vi "Watlow Modbus.vi"(6 "Watlow Present?":bool, 7 "Modbus Mode":T2, 8 "Error IN":errorcluster, 10 "Data Write":sgl format="%#_13g", 11 "Variable":T1) -> (0 "Error OUT":errorcluster, 3 "Data Read":sgl)   [LabVIEW 2019]
uses:
  Modbus Mode.ctl
  Modbus Variable.ctl
  NI Modbus.llb/MB Modbus Command.ctl
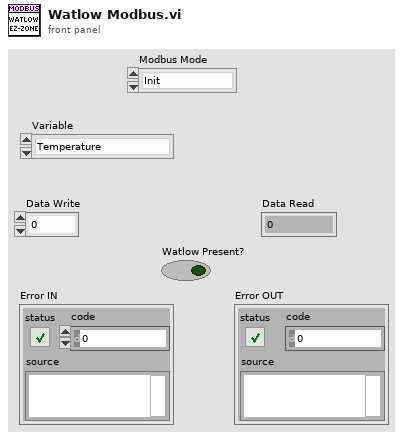
[diagram p1: front panel]
types:
  T1 = typedef "Modbus Variable.ctl" = enum16{"Temperature", "Setpoint"}
  T2 = typedef "Modbus Mode.ctl" = enum16{"Init", "Tank 1 Write", "Tank 2 Write", "Tank 1 Read", "Tank 2 Read", "F4T Write", "F4T Read"}
  T3 = cluster{"Mode":enum16{"RTU", "ASCII"}, "Slave Address":u8}
  T4 = typedef "MB Modbus Command.ctl" = cluster{"Function Code":u8, "Starting Address":u16, "Quantity":u16, "Data":u16[], "Discrete":bool[]}
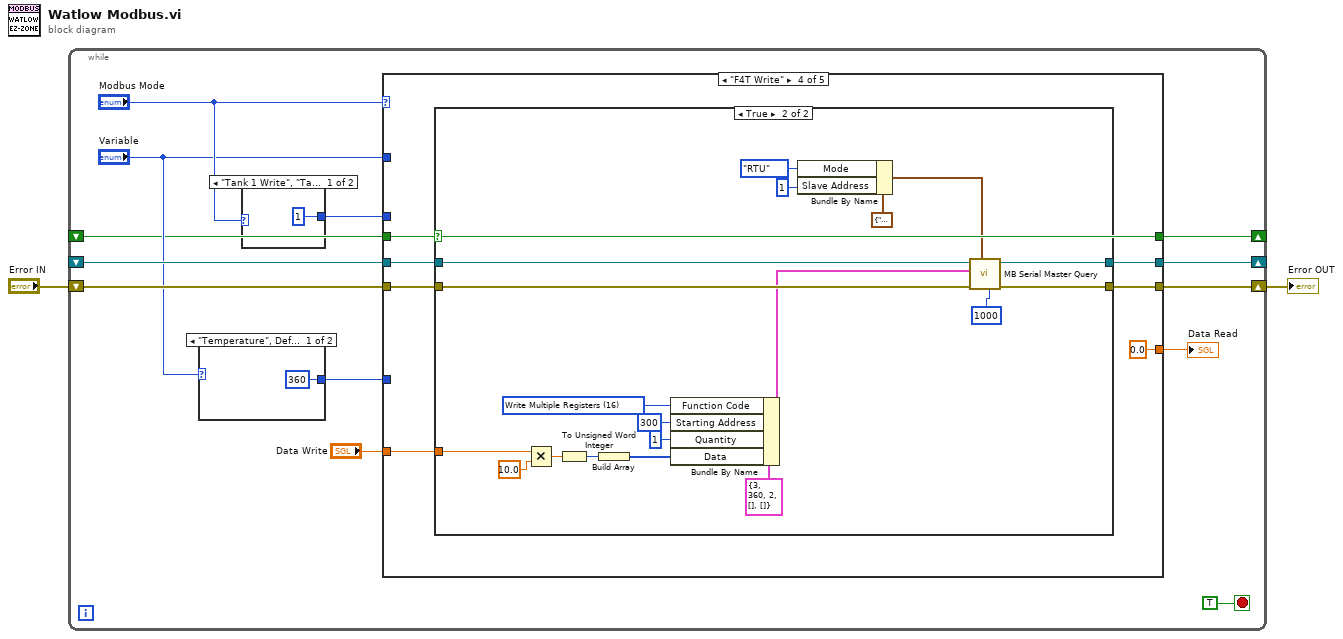
[diagram p0: block diagram]
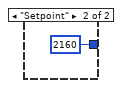
[diagram p2: hidden frame]
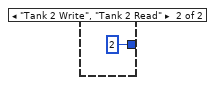
[diagram p3: hidden frame]
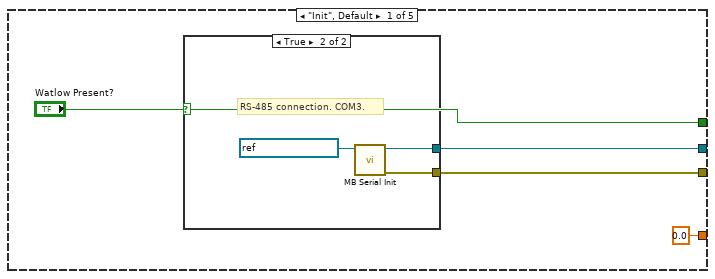
[diagram p4: hidden frame]
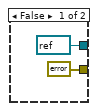
[diagram p5: hidden frame]
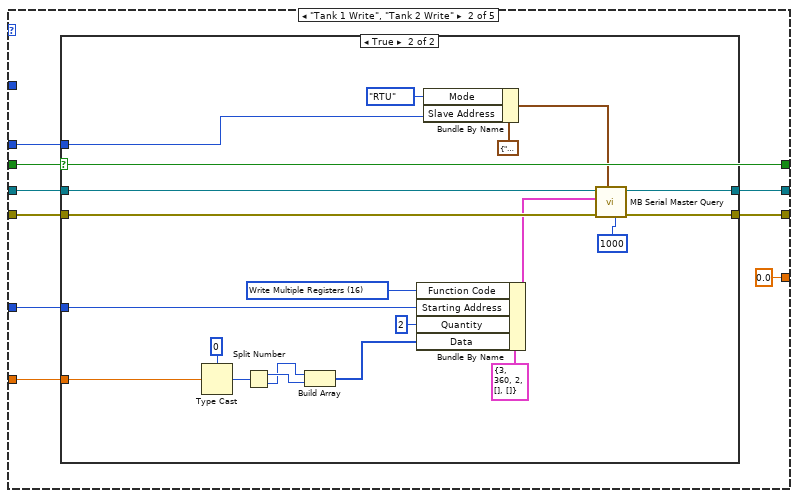
[diagram p6: hidden frame]
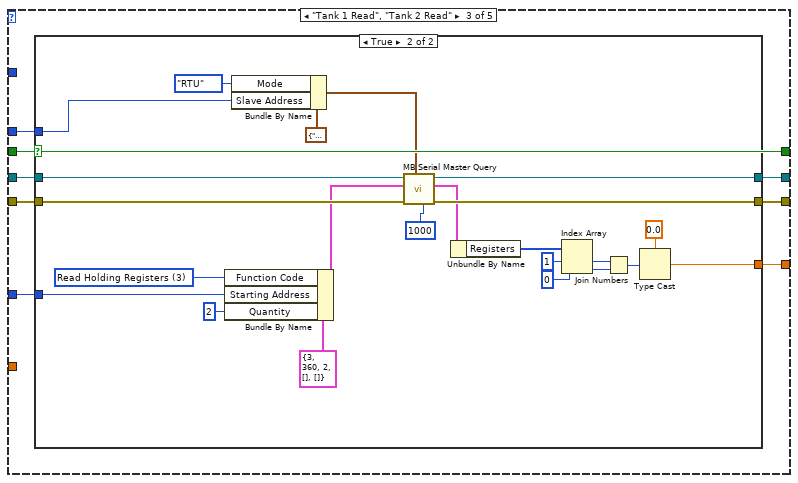
[diagram p8: hidden frame]
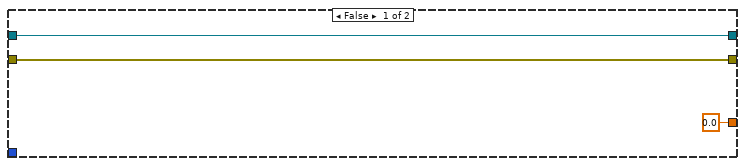
[diagram p9: hidden frame]
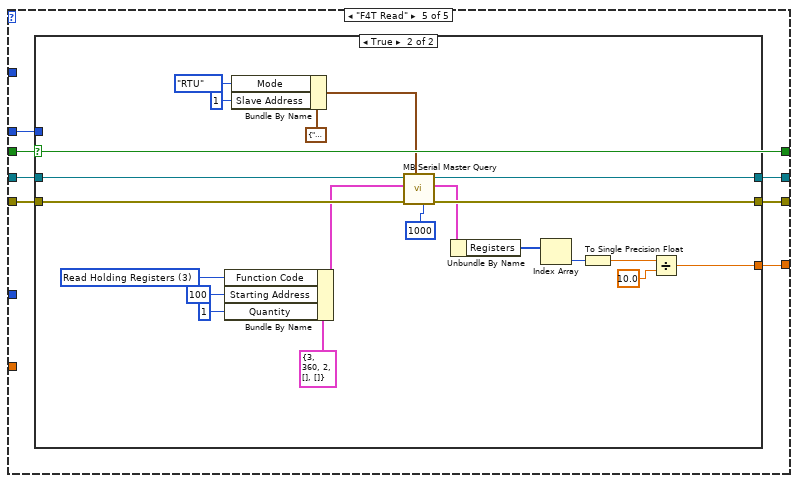
[diagram p11: hidden frame]
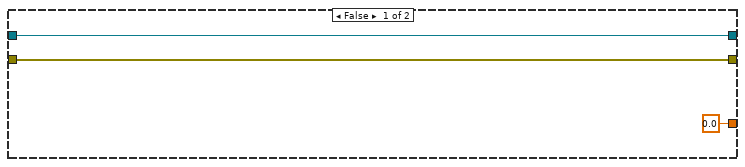
[diagram p12: hidden frame]
diagram:
  n1 = while {
    shift-right: [w14] -> _
    shift-left: _ -> [w12]
    shift-right: [w13] -> w1
    shift-left: "Error IN" -> [w11]
    shift-right: [w6] -> _
    shift-left: _ -> [w5]
    stop <- TRUE stop-if-true
    n2 = case shown="\"Temperature\", Default" "Variable" {
      tunnel: [u16 360 ("Starting Address") u16 2160 ("Starting Address")] -> w8
      frame "Temperature", Default {
      }
      frame "Setpoint" {
      }
    }
    n3 = case shown="\"Tank 1 Write\", \"Tank 1 Read\", Default" "Modbus Mode" {
      tunnel: [u8 1 ("Slave Address") u8 2 ("Slave Address")] -> w9
      frame "Tank 1 Write", "Tank 1 Read", Default {
      }
      frame "Tank 2 Write", "Tank 2 Read" {
      }
    }
    n4 = case shown="\"F4T Write\"" "Modbus Mode" {
      tunnel: "Variable" -> [_ _ _ _ _]
      tunnel: [w23 w36 w66 w96 w124] -> w14
      tunnel: [w22 w35 w65 w97 w123] -> w13
      tunnel: w12 -> [_ w37 w67 w99 w127]
      tunnel: w11 -> [_ w34 w64 w100 w126]
      tunnel: w9 -> [_ w33 w63 _ w128]
      tunnel: w8 -> [_ w32 w62 _ _]
      tunnel: ["Watlow Present?" w31 w61 w98 w125] -> w6
      tunnel: w5 -> [_ w31 w61 w98 w125]
      tunnel: [sgl 0.0 ("single precision float") sgl 0.0 ("single precision float") w60 sgl 0.0 ("single precision float") w122] -> w4
      tunnel: "Data Write" -> [_ w29 _ w94 _]
      frame "Init", Default {
        n5 = case shown="True" "Watlow Present?" {
          tunnel: [refnum<visa-resource-name> refnum ("VISA resource name out") w27] -> w23
          tunnel: [errorcluster {"status"=FALSE, "code"=0, "source"=""} ("error out") w26] -> w22
          frame False {
          }
          frame True {
            # "RS-485 connection. COM3."
            n6 = call "MB Serial Init.vi"("VISA resource name"=refnum<visa-resource-name> "ASRL3::INSTR") -> ("error out"=w26:errorcluster, "VISA resource name out"=w27:refnum<visa-resource-name>)  [unwired: 6 in, 3 out]
          }
        }
      }
      frame "Tank 1 Write", "Tank 2 Write" {
        n7 = case shown="True" w31 {
          tunnel: w37 -> [w39 w59]
          tunnel: [w39 w58] -> w36
          tunnel: [w38 w57] -> w35
          tunnel: w34 -> [w38 w56]
          tunnel: w33 -> [_ w45]
          tunnel: w32 -> [_ w44]
          tunnel: w29 -> [_ w40]
          frame False {
          }
          frame True {
            w53 = u8 16 items=["Read Coils"=1, "Read Discrete Inputs"=2, "Read Holding Registers"=3, "Read Input Registers"=4, "Write Single Coil"=5, "Write Single Register"=6, "Read Exception Status"=7, "Write Multiple Coils"=15, "Write Multiple Registers"=16] ("Function Code")
            n8 = Type Cast(type=u32 0, x=w40) -> (*(type *) &x=w50:u32)
            n9 = Split Number(x=w50) -> (hi(x)=w43:u16, lo(x)=w42:u16)
            n10 = Build Array(w42, w43) -> (w49:u16[])
            n11 = Bundle By Name(cluster=T4 {"Function Code"=3, "Starting Address"=360, "Quantity"=2, "Data"=[], "Discrete"=[]} ("MODBUS Command"), "Function Code"=w53, "Starting Address"=w44, "Quantity"=u16 2, "Data"=w49) -> (w54:T4)
            n12 = Bundle By Name(cluster=T3 {"Mode"=enum."RTU", "Slave Address"=1} ("Serial Parameters"), "Mode"=enum16{"RTU", "ASCII"}."RTU", "Slave Address"=w45) -> (w46:T3)
            n13 = call "MB Serial Master Query.vi"("Timeout"=u32 1000, "Serial Parameters"=w46, "error in (no error)"=w56, "Modbus Command"=w54, "VISA resource name"=w59) -> ("error out"=w57:errorcluster, "VISA resource name out"=w58:refnum<visa-resource-name>)  [unwired: 2 in, 3 out]
          }
        }
      }
      frame "Tank 1 Read", "Tank 2 Read" {
        n14 = case shown="True" w61 {
          tunnel: w67 -> [w70 w93]
          tunnel: [w70 w92] -> w66
          tunnel: [w69 w91] -> w65
          tunnel: w64 -> [w69 w90]
          tunnel: w63 -> [_ w74]
          tunnel: w62 -> [_ w72]
          tunnel: [sgl 0.0 ("single precision float") w71] -> w60
          frame False {
          }
          frame True {
            w87 = u8 3 items=["Read Coils"=1, "Read Discrete Inputs"=2, "Read Holding Registers"=3, "Read Input Registers"=4, "Write Single Coil"=5, "Write Single Register"=6, "Read Exception Status"=7, "Write Multiple Coils"=15, "Write Multiple Registers"=16] ("Function Code")
            n15 = Bundle By Name(cluster=T4 {"Function Code"=3, "Starting Address"=360, "Quantity"=2, "Data"=[], "Discrete"=[]} ("MODBUS Command"), "Function Code"=w87, "Starting Address"=w72, "Quantity"=u16 2) -> (w88:T4)
            n16 = Bundle By Name(cluster=T3 {"Mode"=enum."RTU", "Slave Address"=1} ("Serial Parameters"), "Mode"=enum16{"RTU", "ASCII"}."RTU", "Slave Address"=w74) -> (w84:T3)
            n17 = call "MB Serial Master Query.vi"("Timeout"=u32 1000, "Serial Parameters"=w84, "error in (no error)"=w90, "Modbus Command"=w88, "VISA resource name"=w93) -> ("error out"=w91:errorcluster, "Registers"=w82:cluster{"Registers":u16[], "Discrete":bool[]}, "VISA resource name out"=w92:refnum<visa-resource-name>)  [unwired: 2 in, 2 out]
            n18 = Unbundle By Name(w82) -> ("Registers"=w77:u16[])
            n19 = Index Array(array=w77, index #1=1 ("index"), index #2=0 ("index")) -> (element #1=w78:u16, element #2=w75:u16)
            n20 = Join Numbers(hi=w78, lo=w75) -> ((hi.lo)=w76:u32)
            n21 = Type Cast(type=sgl 0.0 ("single precision float"), x=w76) -> (*(type *) &x=w71:sgl)
          }
        }
      }
      frame "F4T Write" {
        n22 = case shown="True" w98 {
          tunnel: w99 -> [w102 w121]
          tunnel: [w102 w106] -> w96
          tunnel: [w101 w105] -> w97
          tunnel: w100 -> [w101 w120]
          tunnel: w94 -> [_ w110]
          frame False {
          }
          frame True {
            w118 = u8 16 items=["Read Coils"=1, "Read Discrete Inputs"=2, "Read Holding Registers"=3, "Read Input Registers"=4, "Write Single Coil"=5, "Write Single Register"=6, "Read Exception Status"=7, "Write Multiple Coils"=15, "Write Multiple Registers"=16] ("Function Code")
            n23 = Multiply(x=w110, y=sgl 10.0) -> (x*y=w104:sgl)
            n24 = To Unsigned Word Integer(number=w104) -> (unsigned 16bit integer=w108:u16)
            n25 = Build Array(w108) -> (w103:u16[])
            n26 = Bundle By Name(cluster=T4 {"Function Code"=3, "Starting Address"=360, "Quantity"=2, "Data"=[], "Discrete"=[]} ("MODBUS Command"), "Function Code"=w118, "Starting Address"=u16 300, "Quantity"=u16 1, "Data"=w103) -> (w107:T4)
            n27 = Bundle By Name(cluster=T3 {"Mode"=enum."RTU", "Slave Address"=1} ("Serial Parameters"), "Mode"=enum16{"RTU", "ASCII"}."RTU", "Slave Address"=u8 1) -> (w112:T3)
            n28 = call "MB Serial Master Query.vi"("Timeout"=u32 1000, "Serial Parameters"=w112, "error in (no error)"=w120, "Modbus Command"=w107, "VISA resource name"=w121) -> ("error out"=w105:errorcluster, "VISA resource name out"=w106:refnum<visa-resource-name>)  [unwired: 2 in, 3 out]
          }
        }
      }
      frame "F4T Read" {
        n29 = case shown="True" w125 {
          tunnel: w127 -> [w131 w151]
          tunnel: [w131 w150] -> w124
          tunnel: [w130 w149] -> w123
          tunnel: w126 -> [w130 w148]
          tunnel: w128 -> [_ _]
          tunnel: [sgl 0.0 ("single precision float") w132] -> w122
          frame False {
          }
          frame True {
            w145 = u8 3 items=["Read Coils"=1, "Read Discrete Inputs"=2, "Read Holding Registers"=3, "Read Input Registers"=4, "Write Single Coil"=5, "Write Single Register"=6, "Read Exception Status"=7, "Write Multiple Coils"=15, "Write Multiple Registers"=16] ("Function Code")
            n30 = Bundle By Name(cluster=T4 {"Function Code"=3, "Starting Address"=360, "Quantity"=2, "Data"=[], "Discrete"=[]} ("MODBUS Command"), "Function Code"=w145, "Starting Address"=u16 100, "Quantity"=u16 1) -> (w146:T4)
            n31 = Bundle By Name(cluster=T3 {"Mode"=enum."RTU", "Slave Address"=1} ("Serial Parameters"), "Mode"=enum16{"RTU", "ASCII"}."RTU", "Slave Address"=u8 1) -> (w142:T3)
            n32 = call "MB Serial Master Query.vi"("Timeout"=u32 1000, "Serial Parameters"=w142, "error in (no error)"=w148, "Modbus Command"=w146, "VISA resource name"=w151) -> ("error out"=w149:errorcluster, "Registers"=w140:cluster{"Registers":u16[], "Discrete":bool[]}, "VISA resource name out"=w150:refnum<visa-resource-name>)  [unwired: 2 in, 2 out]
            n33 = Unbundle By Name(w140) -> ("Registers"=w139:u16[])
            n34 = Index Array(array=w139) -> (element=w134:u16)  [unwired: 1 in]
            n35 = To Single Precision Float(number=w134) -> (single precision float=w133:sgl)
            n36 = Divide(x=w133, y=sgl 10.0) -> (x/y=w132:sgl)
          }
        }
      }
    }
    "Data Read" <- w4
  }
  "Error OUT" <- w1
